vi "Read_ToProcessEvent.vi"(8 "error in (no error)":errorcluster, 11 "EVE in":refnum<class "EVE.lvclass">) -> (0 "error out":errorcluster, 2 "ToProcessEvent":refnum<user-event>, 3 "EVE out":refnum<class "EVE.lvclass">)   [LabVIEW 2013, in "EVE.lvclass"]
uses:
  EVE.lvclass
  030 - EVENTS/06 - ToProcess/ToProcess.ctl
  030 - EVENTS/06 - ToProcess/ToProcess_EnumCommand.ctl
  EVE.lvclass/EVE.ctl
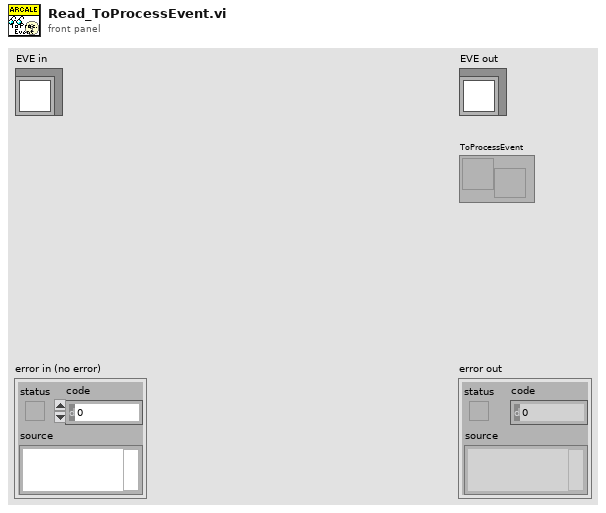
[diagram p1: front panel]
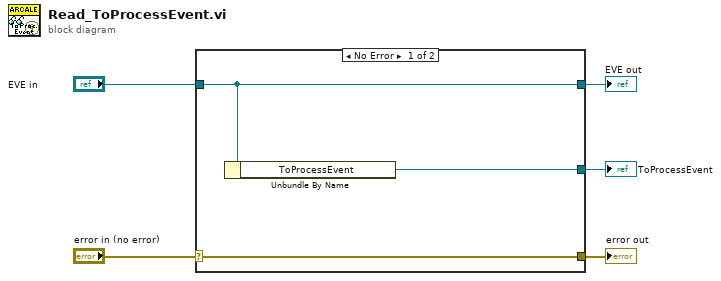
[diagram p0: block diagram]
diagram:
  n1 = case shown="No Error" "error in (no error)" {
    selector: "error in (no error)" -> [w8 w9]
    tunnel: [w8 w9] -> w4
    tunnel: [w7 w10] -> w2
    tunnel: "EVE in" -> [w7 w10]
    tunnel: [w6 _] -> w1
    frame No Error {
      n2 = Unbundle By Name(w7) -> ("ToProcessEvent"=w6:refnum<user-event>)
    }
    frame Error {
    }
  }
  "error out" <- w4
  "EVE out" <- w2
  "ToProcessEvent" <- w1
